vi "Check_if_running.vi"(1 "VI-Pfad":path=path "E:/CryoTUM-Software/16T-Magnet_Ultimate-Control_Version_2-0/LS370Monitor.vi") -> (0 "Running":bool=TRUE)   [LabVIEW 2016]
panel:
  in  "error in":errorcluster
  out "error out":errorcluster
  out "LS 370 Monitor":T1(ring)
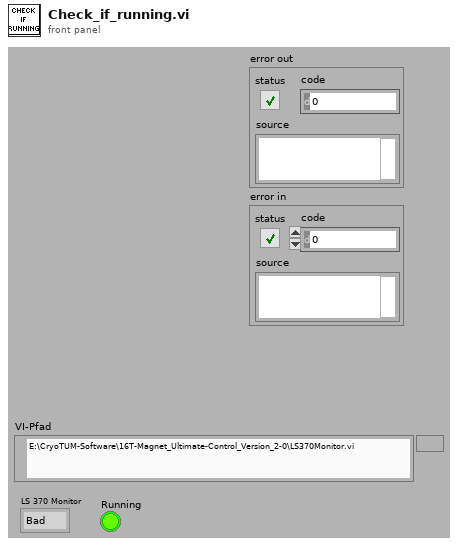
[diagram p1: front panel]
types:
  T1 = enum32{"Bad", "Idle", "Run top level", "Running"}
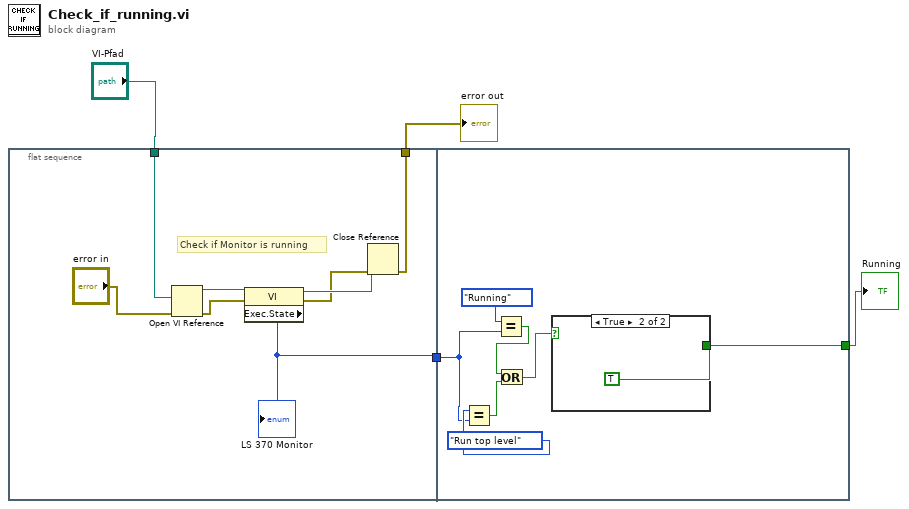
[diagram p0: block diagram]
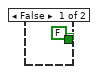
[diagram p2: hidden frame]
diagram:
  n1 = flat-sequence {
    tunnel: [w9] -> w4
    tunnel: "VI-Pfad" -> [w7]
    tunnel: [w6] -> w1
    tunnel: w4 -> [w16]
    tunnel: [w13] -> w2
    frame #0 {
      # "Check if Monitor is running"
      n2 = Open VI Reference(vi path=w7, error in (no error)="error in") -> (vi reference=w8:refnum<vi>, error out=w12:errorcluster)  [unwired: 4 in]
      n3 = property class="VI"(reference=w8, error in=w12) -> (reference out=w11:refnum<vi>, error out=w10:errorcluster, "Exec.State"=w9:T1)
      "LS 370 Monitor" <- w9
      n4 = Close Reference(reference=w11, error in (no error)=w10) -> (error out=w6:errorcluster)
    }
    frame #1 {
      n5 = Equal?(x=T1."Run top level" ("LS 370 Monitor 2"), y=w16) -> (x = y?=w15:bool)
      n6 = Equal?(x=T1."Running" ("LS 370 Monitor 2"), y=w16) -> (x = y?=w18:bool)
      n7 = Or(x=w18, y=w15) -> (x .or. y?=w14:bool)
      n8 = case shown="True" w14 {
        tunnel: [FALSE TRUE] -> w13
        frame False {
        }
        frame True {
        }
      }
    }
  }
  "Running" <- w2
  "error out" <- w1
